vi "setPGAGain.vi"(0 "VISA resource name":refnum<visa-resource-name>, 5 "Bank Sel":bool=TRUE, 7 "Amp Index":u8=7, 9 "Enum":T1(ring), 11 "error in (no error)":errorcluster) -> (4 "VISA resource name out":refnum<visa-resource-name>, 15 "error out":errorcluster)   [LabVIEW 2009]
uses:
  Packet.ctl
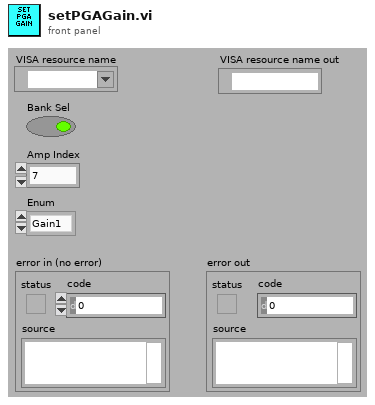
[diagram p1: front panel]
types:
  T1 = enum16{"Gain1", "Gain2", "Gain4", "Gain5", "Gain8", "Gain10", "Gain16", "Gain32", "Gain100", "Gain200", "Gain400", "Gain500", "Gain800", "Gain1000", "Gain1600", "Gain3200"}
  T2 = typedef "Packet.ctl" = cluster{"Length":u8, "Type":u8, "PID":u8, "Data":u8[], "CRC":u8}
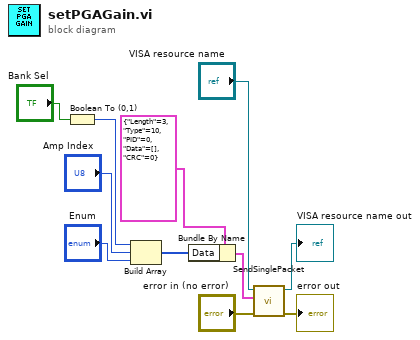
[diagram p0: block diagram]
diagram:
  n1 = Boolean To (0,1)(Boolean="Bank Sel") -> (0, 1=w1:i16)
  n2 = Build Array(w1, "Amp Index", "Enum") -> (w5:u16[])
  n3 = Bundle By Name(cluster=T2 {"Length"=3, "Type"=10, "PID"=0, "Data"=[], "CRC"=0} ("Transmit"), "Data"=w5) -> (w11:T2)
  n4 = call "SendSinglePacket.vi"("error in (no error)"="error in (no error)", "Transmit"=w11, "VISA resource name"="VISA resource name") -> ("error out"=→"error out":errorcluster, "VISA resource name out"=→"VISA resource name out":refnum<visa-resource-name>)  [unwired: 6 in, 1 out]
